vi "GetScale.vi"(11 "AI in":refnum<class "AI.lvclass">) -> (2 "Scale_PiecedLinear.lvclass":refnum<class "Scale_PiecedLinear.lvclass">)   [LabVIEW 2019, in "AI.lvclass"]
uses:
  AI.lvclass
  PiecedLinearScale_class/Scale_PiecedLinear.lvclass
  AI.lvclass/AI.ctl
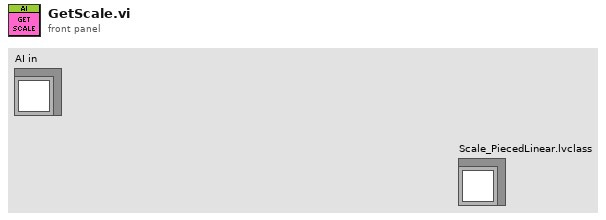
[diagram p1: front panel]
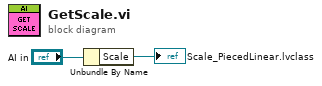
[diagram p0: block diagram]
diagram:
  n1 = Unbundle By Name("AI in") -> ("Scale"=→"Scale_PiecedLinear.lvclass":refnum<class "Scale_PiecedLinear.lvclass">)
